vi "Configure_Trigger_Source.vi"(8 "error in (no error)":errorcluster, 9 "ON/OFF TRIGGER":bool, 11 "VISA resource name":refnum<visa-resource-name>) -> (0 "error out":errorcluster, 3 "VISA resource name out":refnum<visa-resource-name>)   [LabVIEW 2023]
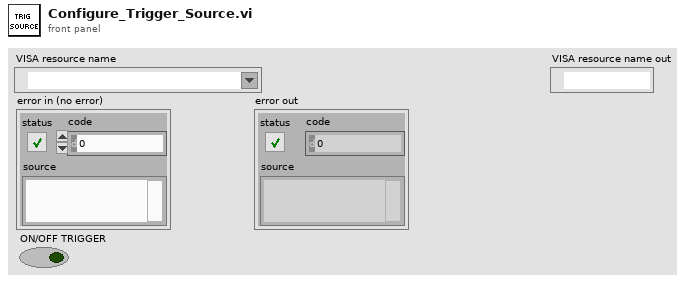
[diagram p1: front panel]
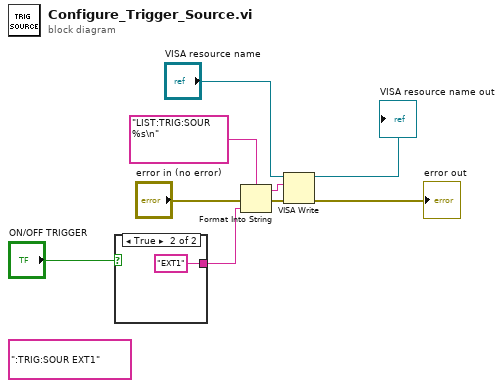
[diagram p0: block diagram]
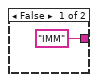
[diagram p2: hidden frame]
diagram:
  (unwired) ":TRIG:SOUR EXT1" ("string")
  n1 = case shown="True" "ON/OFF TRIGGER" {
    tunnel: ["IMM" "EXT1"] -> w2
    frame False {
    }
    frame True {
    }
  }
  n2 = Format Into String(format string="LIST:TRIG:SOUR  %s\n" ("string"), error in="error in (no error)", w2) -> (resulting string=w5:string, error out=w3:errorcluster)  [unwired: 1 in]
  n3 = VISA Write(VISA resource name="VISA resource name", write buffer=w5, error in (no error)=w3) -> (VISA resource name out=→"VISA resource name out":refnum<visa-resource-name>, error out=→"error out":errorcluster)  [unwired: 1 out]
